vi "PWM Servo FPGA Solution.vi"() -> ()   [LabVIEW 2012]
doc: "This VI shows an example of how to implement a closed loop position move using the NI 9505. The position loop is implemented using PID. The output of the loop is used as the command for the current loop, which then sets the PWM duty cycle for the motor. This example assumes that an encoder is connected for position and velocity feedback. This example does not implement advanced motion features such as trajectory generation and splining."
uses:
  <vilib>/LabVIEW Targets/FPGA/cRIO/cRIO-9505/controls.llb/_nicrio_cRIO-9505_DriveStatus.ctl
  <vilib>/Platform/TimedLoop/XDataNode/timing_clust.ctl
  <vilib>/Platform/TimedLoop/XDataNode/nitl_modes.ctl
  <vilib>/Platform/TimedLoop/XDataNode/wakeup.ctl
  <vilib>/LabVIEW Targets/FPGA/cRIO/cRIO-9505/controls.llb/_nicrio_cRIO-9505_DriveDirection.ctl
  Instance           1 55Saved   Position Control (closed loop) - NI 9505 (FPGA) .vi
  <vilib>/rvi/Emulation/niFpgaSctlEmulationRegisterWithScheduler.vi
  <vilib>/rvi/Emulation/niFpgaSctlEmulationScheduler.vi
  <vilib>/rvi/eio/common/nirviEmuTemplateMethod_errors.vi
  Instance           2 55Saved   Position Control (closed loop) - NI 9505 (FPGA) .vi
  Instance           3 55Saved   Position Control (closed loop) - NI 9505 (FPGA) .vi
  <vilib>/rvi/eio/common/nirviEmuTemplatePropertyGet_noerrors.vi
  Instance           4 55Saved   Position Control (closed loop) - NI 9505 (FPGA) .vi
  <vilib>/Platform/TimedLoop/XDataNode/XDataNode.xnode
  <vilib>/eio/EIONode/EIONode.xnode
  <vilib>/addons/control/pid/fpga.llb/XNode/niFpgaPID.xnode
  <vilib>/eio/EIOMethodNode/EIOMethodNode.xnode
  <vilib>/eio/EIOPropertyNode/EIOPropertyNode.xnode
  <vilib>/Platform/TimedLoop/XDataNode/XDNodeRunTimeDep.lvlib
  <vilib>/rvi/eio/common/nirviEmuTemplatePropertyGet_errors.vi
  <vilib>/rvi/eio/common/nirviEmuTemplatePropertySet_errors.vi
  <vilib>/rvi/eio/common/nirviEmuTemplatePropertySet_noerrors.vi
panel:
  out "Go forward?":bool
  out "Coerced Current":i16
  out "Current PID output":i16
  out "Current Feedback":i16
  in  "PID gains":T1={"proportional gain (Kc)"=20.0, "integral gain (Kc*Ts/Ti)"=10.0, "derivative gain (Kc*Td/Ts)"=0.0}
  in  "Current Limit":i16=806
  in  "Current Loop Rate (usec)":u16=50
  in  "Position PID Gains":T2={"Kp"=50, "Kd"=1000, "Ki"=0, "ILim"=1000, "Kv"=0, "Vff"=0, "Aff"=0, "Td"=0}
  out "Vsup Present":bool
  out "Drive Fault":bool
  out "Drive Status":T3=enum."Disabled"
  out "Temp Fault":bool
  in  "Enable\nDrive":bool
  in  "Disable\nDrive":bool
  in  "Reset Position":bool
  in  "Reset Position Value":i32
  out "Encoder Position":i32
  out "ticks/count":u32
  out "Index (Z) Position":i32
  out "counts (no reset)":i32
  in  "Position Loop  Rate (usec)":u16=250
  in  "Position Error Limit":i16=32767
  out "Position Error Read":i16
  out "Position Error Status":bool
  in  "Position Setpoint":i32 caption="Setpoint"
  out "Trig AI":bool
  out "Current Loop Output":i16
  out "Current Command":i16
  # "These parameters control the response of the position loop. Position Setpoint is the desired position to go to. Position Error Limit is the maximum allowed error the setpoint and actual position returned by the encoder loop."
  # "These parameters control the response\nof the current loop. The current limit is the \nmaximum current allowed."
  # "Use \"Enable Drive\" and \"Disable Drive\" to \nturn start and stop motor"
  # "Current Loop Parameters"
  # "Enter Position Setpoint\nto manually move the\nmotor"
  # "These status controls/indicators are used to enable/disable the drive and read fault information."
  # "Feedback for Troubleshooting"
  # "Use the Reset Position control to reset the quadrature count to the value in Reset Position Value."
  # "Drive Status"
  # "Encoder Parameters"
  # "Position Loop Parameters"
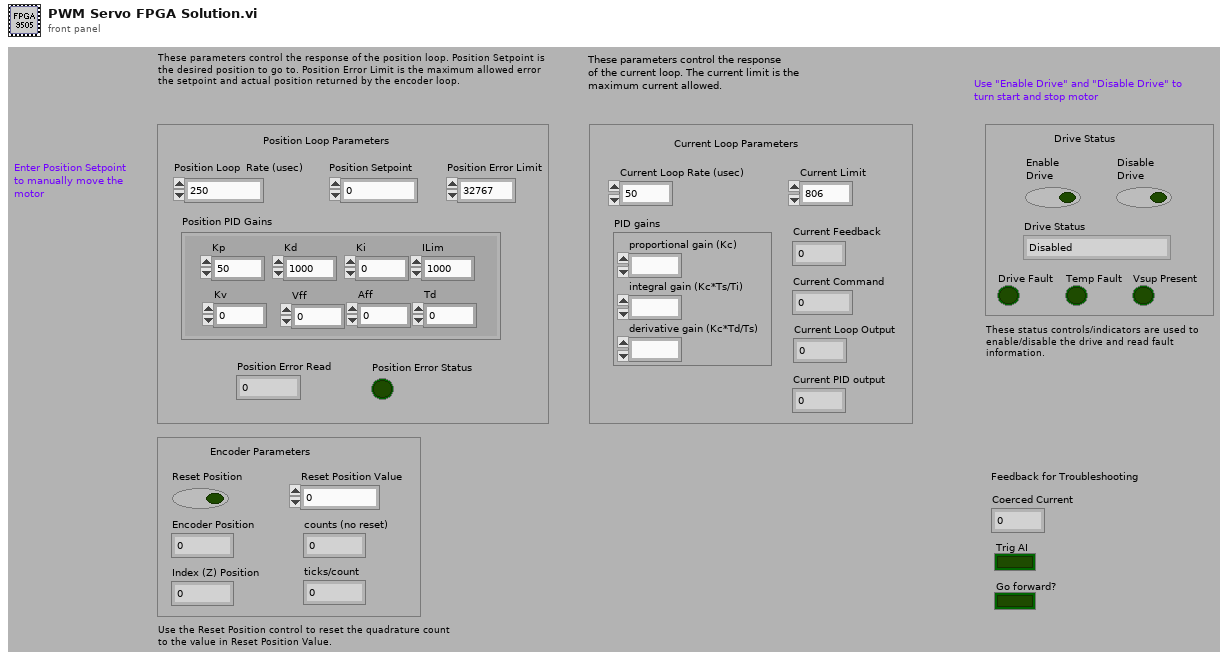
[diagram p1: front panel]
types:
  T1 = cluster{"proportional gain (Kc)":fxp<+/-,16,8>, "integral gain (Kc*Ts/Ti)":fxp<+/-,16,8>, "derivative gain (Kc*Td/Ts)":fxp<+/-,16,8>}
  T2 = cluster{"Kp":i16, "Kd":i16, "Ki":i16, "ILim":i16, "Kv":i16, "Vff":i16, "Aff":i16, "Td":i16}
  T3 = typedef "_nicrio_cRIO-9505_DriveStatus.ctl" = enum8{"Enabled", "Disabled", "Disabled by Drive Fault", "Disabled by Temp. Fault", "Disabled by E-Stop", "Unknown"}
  T4 = typedef "XDNodeRunTimeDep.lvlib/timing_clust.ctl" = cluster{"Expected End [f-1]":u64, "Actual End [f-1]":u64, "Finished Late? [f-1]":bool, "Expected End [i-1]":u64, "Actual End [i-1]":u64, "Finished Late? [i-1]":bool, "Expected Start [i]":u64, "Actual Start [i]":u64, "Expected Start [f]":u64, "Actual Start [f]":u64, "Source Name":string, "Structure Name":string, "Period":i64, "Deadline":i64, "Offset":i64, "Start":i64, "Priority":i32, "Timeout":i32, "Mode":T5, "Wakeup Reason":T6, "Error":errorcluster, "Source Type":string, "Secondary Source Type":string, "Global End Time":u64, "Global Start Time":u64, "Frame Duration":u64, "Iteration Duration":u64, "Assigned CPU":i32, "I/O Scan Engine Mode":u32}
  T5 = typedef "XDNodeRunTimeDep.lvlib/nitl_modes.ctl" = enum32{"No Change", "Process missed periods, maintain original phase", "Discard missed periods, maintain original phase", "Process missed periods, ignore original phase", "Discard missed periods, ignore original phase"}
  T6 = typedef "XDNodeRunTimeDep.lvlib/wakeup.ctl" = enum32{"Normal", "Aborted", "Asynchronous wakeup", "Timing source error", "Timed loop error", "Timeout"}
  T7 = cluster{"proportional gain (Kc)":i16, "integral gain (Kc*Ts/Ti)":i16, "derivative gain (Kc*Td/Ts)":i16}
  T8 = typedef "_nicrio_cRIO-9505_DriveDirection.ctl" = enum8{"Clockwise", "Counterclockwise"}
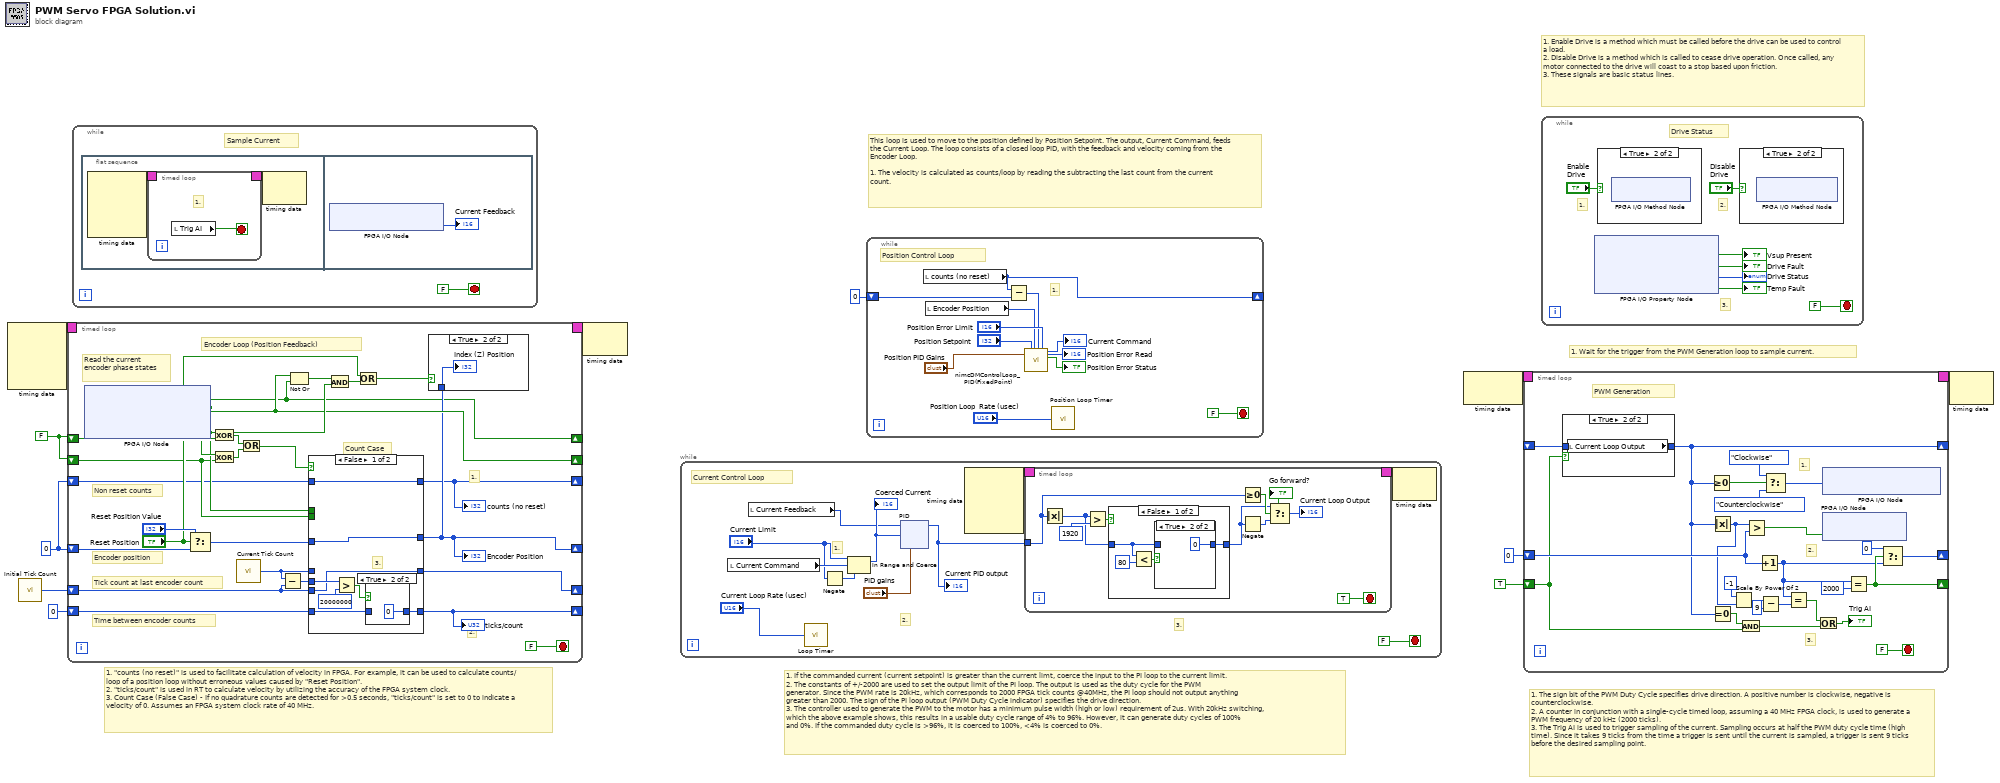
[diagram p0: block diagram]
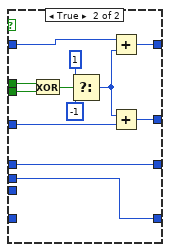
[diagram p4: hidden frame]
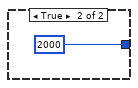
[diagram p7: hidden frame]
diagram:
  w1 = 0 ("Reset Position Value")
  w4 = FALSE ("Encoder Phase A")
  # "1. \"counts (no reset)\" is used to facilitate calculation of velocity in FPGA. For example, it can be used to calculate counts/loop of a position loop without erroneous values caused by \"Reset Position\". \n2. \"ticks/count\" is used in RT to calculate velocity by utilizing the accuracy of the FPGA system clock.\n3. Count Case (False Case) - If no quadrature counts are detected for >0.5 seconds, \"ticks/count\" is set to 0 to indicate a velocity of 0. Assumes an FPGA system clock rate of 40 MHz."
  # "1. Enable Drive is a method which must be called before the drive can be used to control a load.\n2. Disable Drive is a method which is called to cease drive operation. Once called, any motor connected to the drive will coast to a stop based upon friction.\n3. These signals are basic status lines."
  # "This loop is used to move to the position defined by Position Setpoint. The output, Current Command, feeds the Current Loop. The loop consists of a closed loop PID, with the feedback and velocity coming from the Encoder Loop.\n\n1. The velocity is calculated as counts/loop by reading the subtracting the last count from the current count."
  # "1. The sign bit of the PWM Duty Cycle specifies drive direction. A positive number is clockwise, negative is counterclockwise. \n2. A counter in conjunction with a single-cycle timed loop, assuming a 40 MHz FPGA clock, is used to generate a PWM frequency of 20 kHz (2000 ticks).\n3. The Trig AI is used to trigger sampling of the current. Sampling occurs at half the PWM duty cycle time (high time). Since it takes 9 ticks from the time a trigger is sent until the current is sampled, a trigger is sent 9 ticks before the desired sampling point."
  # "1. Wait for the trigger from the PWM Generation loop to sample current."
  # "1. If the commanded current (current setpoint) is greater than the current limt, coerce the input to the PI loop to the current limit.\n2. The constants of +/-2000 are used to set the output limit of the PI loop. The output is used as the duty cycle for the PWM\ngenerator. Since the PWM rate is 20kHz, which corresponds to 2000 FPGA tick counts @40MHz, the PI loop should not output anything\ngreater than 2000. The sign of the PI loop output (PWM Duty Cycle indicator) specifies the drive direction.\n3. The controller used to generate the PWM to the motor has a minimum pulse width (high or low) requirement of 2us. With 20kHz switching,\nwhich the above example shows, this results in a usable duty cycle range of 4% to 96%. However, it can generate duty cycles of 100%\nand 0%. If the commanded duty cycle is >96%, it is coerced to 100%, <4% is coerced to 0%."
  n1 = node-c288() -> (w6:T4)  [unwired: 4 out]
  n2 = call "Initial Tick Count"() -> ("Tick Count(Ticks)"=w3:u32)
  n3 = timed-loop {
    shift-right: [w18] -> _
    shift-left: w4 -> [w36]
    shift-right: [w24] -> _
    shift-left: w4 -> [w17]
    shift-right: [w20] -> _
    shift-left: w1 -> [w33]
    shift-right: [w29] -> _
    shift-left: w3 -> [w13]
    shift-right: [w28] -> _
    shift-left: u32 0 -> [w27]
    timing: w6 -> [_]
    timing-out: [_] -> w5
    shift-right: [w15] -> _
    shift-left: w1 -> [w16]
    stop <- FALSE stop-if-true
    # "Count Case"
    # "Encoder Loop (Position Feedback)"
    # "2."
    # "1."
    # "Read the current\nencoder phase states"
    # "Non reset counts"
    # "Encoder position"
    # "Time between encoder counts"
    # "Tick count at last encoder count"
    n4 = xnode "FPGA I/O Node"() -> ("Mod7/Encoder Phase A"=w18:bool, "Mod7/Encoder Phase B"=w24:bool, "Mod7/Encoder Index"=w25:bool)  [unwired: 3 in, 3 out]
    n5 = Select(t="Reset Position Value", s="Reset Position", f=w33) -> (s? t:f=w31:i32)
    n6 = Exclusive Or(1:w36, 2:w18) -> (0:w35:bool)
    n7 = Exclusive Or(1:w17, 2:w24) -> (0:w34:bool)
    n8 = call "Current Tick Count"() -> ("Tick Count(Ticks)"=w14:u32)
    n9 = Or(x=w35, y=w34) -> (x .or. y?=w32:bool)
    n10 = Subtract(x=w14, y=w13) -> (x-y=w12:u32)
    n11 = Not Or(1:w18, 2:w24) -> (0:w22:bool)
    n12 = case shown="False" w32 {
      tunnel: [w45 w53] -> w20
      tunnel: w31 -> [w45 w59]
      tunnel: w14 -> [_ w49]
      tunnel: [w40 w49] -> w29
      tunnel: w13 -> [w40 _]
      tunnel: [w38 w48] -> w28
      tunnel: w27 -> [w39 _]
      tunnel: w18 -> [_ w55]
      tunnel: w17 -> [_ w54]
      tunnel: [w44 w51] -> w15
      tunnel: w16 -> [w44 w50]
      tunnel: w12 -> [w41 w48]
      frame False {
        # "3."
        n13 = Greater?(x=w41, y=20000000 ("x")) -> (0:w42:bool)
        n14 = case shown="True" w42 {
          tunnel: [w46 u32 0] -> w38
          tunnel: w39 -> [w46 _]
          frame False {
          }
          frame True {
          }
        }
      }
      frame True {
        n15 = Exclusive Or(1:w54, 2:w55) -> (0:w56:bool)
        n16 = Select(t=1 ("16 bit"), s=w56, f=-1 ("16 bit")) -> (s? t:f=w52:i32)
        n17 = Add(x=w50, y=w52) -> (x+y=w51:i32)
        n18 = Add(x=w52, y=w59) -> (x+y=w53:i32)
      }
    }
    "Encoder Position" <- w20
    "ticks/count" <- w28
    "counts (no reset)" <- w15
    n19 = And(x=w22, y=w25) -> (x .and. y?=w23:bool)
    n20 = Or(x="Reset Position", y=w23) -> (x .or. y?=w21:bool)
    n21 = case shown="True" w21 {
      tunnel: w20 -> [_ w37]
      frame False {
      }
      frame True {
        "Index (Z) Position" <- w37
      }
    }
  }
  n22 = while {
    stop <- FALSE stop-if-true
    # "Sample Current"
    n23 = flat-sequence {
      frame #0 {
        n24 = node-c288() -> (w64:T4)  [unwired: 4 out]
        n25 = timed-loop {
          timing: w64 -> [_]
          timing-out: [_] -> w63
          stop <- w65 stop-if-true
          # "1."
          n26 = local read "Trig AI"() -> (w65:bool)
        }
        n27 = node-c288(w63) -> ()  [unwired: 1 out]
      }
      frame #1 {
        n28 = xnode "FPGA I/O Node"() -> ("Mod7/Current Sense"=→"Current Feedback":i16)  [unwired: 1 in, 1 out]
      }
    }
  }
  n29 = node-c288(w5) -> ()  [unwired: 1 out]
  n30 = while {
    stop <- FALSE stop-if-true
    # "3."
    # "2."
    # "1."
    # "Current Control Loop"
    n31 = local read "Current Command"() -> (w77:i16)
    n32 = local read "Current Feedback"() -> (w71:i16)
    n33 = call "Loop Timer"("Count(uSec)"="Current Loop Rate (usec)") -> ()  [unwired: 1 out]
    n34 = Negate(x="Current Limit") -> (-x=w78:i16)
    n35 = In Range and Coerce(upper limit="Current Limit", x=w77, lower limit=w78) -> (coerced(x)=w74:i16)  [unwired: 1 out]
    "Coerced Current" <- w74
    n36 = xnode "PID"("process variable"=w71, "setpoint"=w74, "PID gains"="PID gains") -> ("output"=w72:i16)  [unwired: 2 in]
    "Current PID output" <- w72
    n37 = node-c288() -> (w80:T4)  [unwired: 4 out]
    n38 = timed-loop {
      timing: w80 -> [_]
      timing-out: [_] -> w79
      tunnel: w72 -> [w112]
      stop <- TRUE stop-if-true
      n39 = Absolute Value(x=w112) -> (abs(x)=w113:i16)
      n40 = Greater?(x=w113, y=i16 1920 ("upper limit")) -> (0:w115:bool)
      n41 = case shown="False" w115 {
        tunnel: [w121 i16 2000 ("upper limit")] -> w114
        tunnel: w113 -> [w119 _]
        frame False {
          n42 = Less?(x=w119, y=i16 80 ("lower limit")) -> (x < y?=w120:bool)
          n43 = case shown="True" w120 {
            tunnel: [w123 i16 0 ("upper limit")] -> w121
            tunnel: w119 -> [w123 _]
            frame False {
            }
            frame True {
            }
          }
        }
        frame True {
        }
      }
      n44 = Greater Or Equal To 0?(x=w112) -> (x >= 0?=w118:bool)
      "Go forward?" <- w118
      n45 = Negate(x=w114) -> (-x=w117:i16)
      n46 = Select(t=w114, s=w118, f=w117) -> (s? t:f=→"Current Loop Output":i16)
    }
    n47 = node-c288(w79) -> ()  [unwired: 1 out]
  }
  n48 = while "Position Control Loop" {
    shift-right: [w134] -> _
    shift-left: 0 ("Encoder Position") -> [w136]
    stop <- FALSE stop-if-true
    # "1."
    # "Position Control Loop"
    n49 = local read "counts (no reset)"() -> (w134:i32)
    n50 = local read "Encoder Position"() -> (w131:i32)
    n51 = Subtract(x=w134, y=w136) -> (x-y=w135:i32)
    n52 = call "nimcDMControlLoop_PID(FixedPoint).vi"("PID Gains"="Position PID Gains", "Setpoint"="Position Setpoint", "Position Feedback"=w131, "Velocity Feedback"=w135, "Position Error Limit"="Position Error Limit") -> ("Output"=→"Current Command":i16, "Position Error Read"=→"Position Error Read":i16, "Position Error Status"=→"Position Error Status":bool)  [unwired: 2 in, 10 out]
    n53 = call "Position Loop Timer"("Count(uSec)"="Position Loop  Rate (usec)") -> ()  [unwired: 1 out]
  }
  n54 = node-c288() -> (w11:T4)  [unwired: 1 out]
  n55 = timed-loop {
    timing: w11 -> [_]
    timing-out: [_] -> w10
    shift-right: [w162] -> _
    shift-left: i16 0 -> [w165]
    shift-right: [w161] -> _
    shift-left: TRUE -> [w158]
    shift-right: [w145] -> _
    shift-left: _ -> [w160]
    stop <- FALSE stop-if-true
    # "3."
    # "2."
    # "1."
    # "PWM Generation"
    n56 = case shown="True" w158 {
      tunnel: [w166 w167] -> w145
      tunnel: w160 -> [w166 _]
      frame False {
      }
      frame True {
        n57 = local read "Current Loop Output"() -> (w167:i16)
      }
    }
    n58 = Greater Or Equal To 0?(x=w145) -> (x >= 0?=w154:bool)
    n59 = Absolute Value(x=w145) -> (abs(x)=w143:i16)
    n60 = Equal To 0?(x=w145) -> (x = 0?=w159:bool)
    n61 = Scale By Power Of 2(n=i8 -1, x=w143) -> (x*2^n=w147:i16)
    n62 = And(x=w159, y=w158) -> (x .and. y?=w155:bool)
    n63 = Greater?(x=w143, y=w165) -> (0:w151:bool)
    n64 = Increment(x=w165) -> (x+1=w157:i16)
    n65 = Subtract(x=w147, y=i8 9) -> (x-y=w146:i16)
    n66 = Select(t=_nicrio_cRIO-9505_DriveDirection."Clockwise" ("Drive Direction"), s=w154, f=_nicrio_cRIO-9505_DriveDirection."Counterclockwise" ("Drive Direction")) -> (s? t:f=w150:T8)
    n67 = Equal?(x=w157, y=w146) -> (x = y?=w156:bool)
    n68 = Or(x=w156, y=w155) -> (x .or. y?=→"Trig AI":bool)
    n69 = xnode "FPGA I/O Node"("Mod7/Drive Direction"=w150) -> ()  [unwired: 1 in, 1 out]
    n70 = xnode "FPGA I/O Node"("Mod7/Motor"=w151) -> ()  [unwired: 1 in, 1 out]
    n71 = Equal?(x=w157, y=i16 2000) -> (x = y?=w161:bool)
    n72 = Select(t=i16 0, s=w161, f=w157) -> (s? t:f=w162:i16)
  }
  n73 = while {
    stop <- FALSE stop-if-true
    # "Drive Status"
    # "3."
    # "2."
    # "1."
    n74 = xnode "FPGA I/O Property Node"() -> ("Vsup Present"=→"Vsup Present":bool, "Drive Fault"=→"Drive Fault":bool, "Drive Status"=→"Drive Status":T3, "Over Temperature Fault"=→"Temp Fault":bool)  [unwired: 1 in, 1 out]
    n75 = case shown="True" "Enable\nDrive" {
      frame False {
      }
      frame True {
        n76 = xnode "FPGA I/O Method Node"() -> ()  [unwired: 1 in, 1 out]
      }
    }
    n77 = case shown="True" "Disable\nDrive" {
      frame False {
      }
      frame True {
        n78 = xnode "FPGA I/O Method Node"() -> ()  [unwired: 1 in, 1 out]
      }
    }
  }
  n79 = node-c288(w10) -> ()  [unwired: 1 out]
